vi "_PC_Pub_ExpCondiValue_Laser.vi"(2 "error in (no error)":errorcluster, 3 "expCondiVariant":variant) -> (0 "error out":errorcluster, 1 "laserParam":string)   [LabVIEW 2018]
uses:
  <vilib>/Utility/error.llb/Error Cluster From Error Code.vi
  <vilib>/ErrorRing/Error Ring.xnode
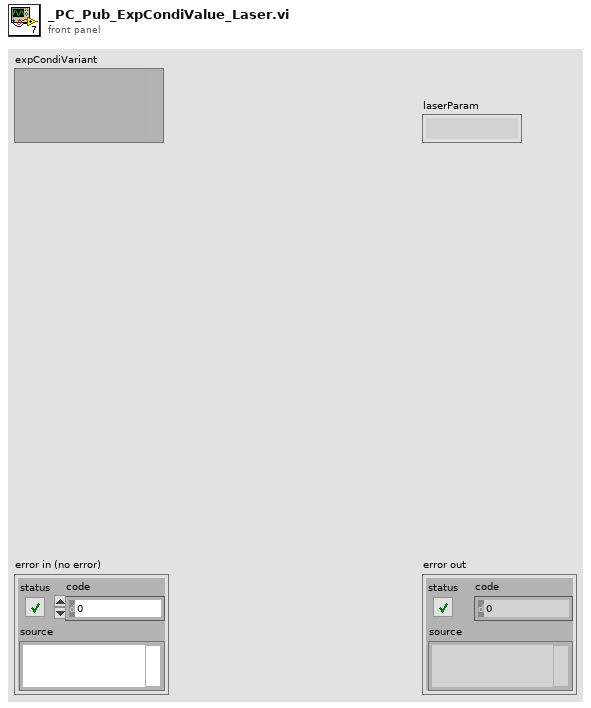
[diagram p1: front panel]
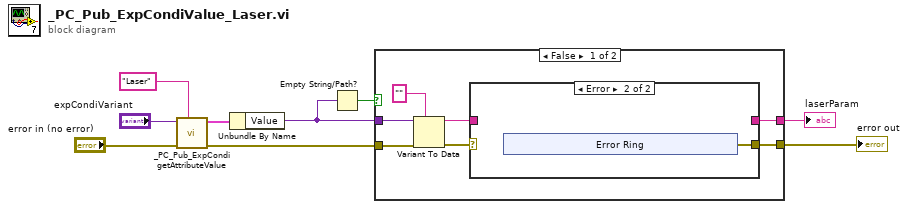
[diagram p0: block diagram]
diagram:
  n1 = call "_PC_Pub_ExpCondi getAttributeValue.vi"("attrName"="Laser", "error in (no error)"="error in (no error)", "expCondiVariant"="expCondiVariant") -> ("error out"=w7:errorcluster, "attrValue"=w9:cluster{"Label":string, "Value":variant})  [unwired: 7 in]
  n2 = Unbundle By Name(w9) -> ("Value"=w2:variant)
  n3 = Empty String/Path?(string/path=w2) -> (empty?=w1:bool)
  n4 = case shown="False" w1 {
    tunnel: w7 -> [w16 w24]
    tunnel: [w13 w24] -> w5
    tunnel: [w11 _] -> w3
    tunnel: w2 -> [w10 _]
    frame False {
      n5 = Variant To Data(error in=w16, type="", Variant=w10) -> (data=w14:string, error out=w15:errorcluster)
      n6 = case shown="Error" w15 {
        selector: w15 -> [w17 _]
        tunnel: w14 -> [w18 _]
        tunnel: [w18 _] -> w11
        tunnel: [w17 w19] -> w13
        frame No Error {
        }
        frame Error {
          n7 = xnode "Error Ring"() -> ("error out"=w19:errorcluster)
        }
      }
    }
    frame True {
    }
  }
  "laserParam" <- w3
  "error out" <- w5
